vi "Auton Edit Queue.vi"(10 "Add?":bool, 11 "Delete?":bool) -> ()   [LabVIEW 2016]
uses:
  Robot Global Data.vi
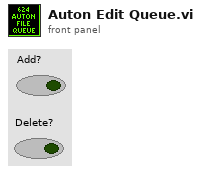
[diagram p1: front panel]
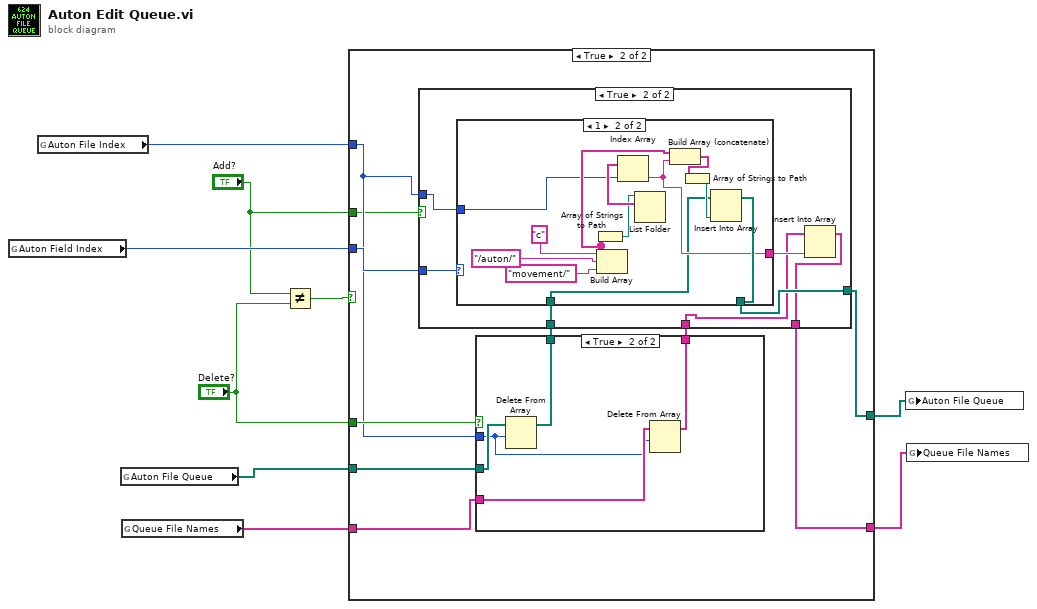
[diagram p0: block diagram]
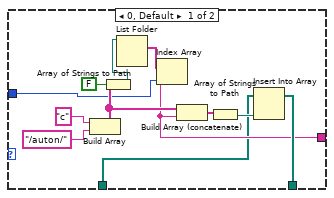
[diagram p5: hidden frame]
diagram:
  n1 = global read "Robot Global Data.vi" "Auton Field Index"() -> (w7:i32)
  n2 = global read "Robot Global Data.vi" "Auton File Index"() -> (w8:i32)
  n3 = global read "Robot Global Data.vi" "Auton File Queue"() -> (w6:path[])
  n4 = global read "Robot Global Data.vi" "Queue File Names"() -> (w5:string[])
  n5 = Not Equal?(x="Add?", y="Delete?") -> (x != y?=w9:bool)
  n6 = case shown="True" w9 {
    tunnel: w8 -> [_ w13]
    tunnel: w7 -> [_ w14]
    tunnel: [w11 w17] -> w4
    tunnel: w6 -> [w11 w21]
    tunnel: [w10 w15] -> w3
    tunnel: w5 -> [w10 w19]
    tunnel: "Delete?" -> [_ w20]
    tunnel: "Add?" -> [_ w12]
    frame False {
    }
    frame True {
      n7 = case shown="True" w20 {
        tunnel: w21 -> [w23 w28]
        tunnel: w19 -> [w22 w27]
        tunnel: [w23 w26] -> w18
        tunnel: [w22 w25] -> w16
        tunnel: w13 -> [_ w24]
        frame False {
        }
        frame True {
          n8 = Delete From Array(array=w28, length=w24) -> (array with subset deleted=w26:path[])  [unwired: 1 in, 1 out]
          n9 = Delete From Array(array=w27, length=w24) -> (array with subset deleted=w25:string[])  [unwired: 1 in, 1 out]
        }
      }
      n10 = case shown="True" w12 {
        tunnel: w18 -> [w30 w35]
        tunnel: [w30 w34] -> w17
        tunnel: w16 -> [w29 w32]
        tunnel: [w29 w31] -> w15
        tunnel: w14 -> [_ w37]
        tunnel: w13 -> [_ w36]
        frame False {
        }
        frame True {
          n11 = case shown="1" w37 {
            tunnel: [w47 w59] -> w34
            tunnel: [w40 w52] -> w33
            tunnel: w36 -> [w38 w50]
            tunnel: w35 -> [w39 w51]
            frame 0, Default {
              n12 = Build Array("c", "/auton/") -> (w42:string[])
              n13 = Array of Strings to Path(0:w42, 1:FALSE ("relative")) -> (2:w44:path)
              n14 = List Folder(path=w44) -> (filenames=w49:string[])  [unwired: 3 in, 3 out]
              n15 = Index Array(array=w49, index=w38) -> (element=w40:string)
              n16 = Build Array (concatenate)(w42, w40) -> (w41:string[])
              n17 = Array of Strings to Path(0:w41) -> (2:w48:path)  [unwired: 1 in]
              n18 = Insert Into Array(array=w39, new element=w48) -> (w47:path[])  [unwired: 1 in]
            }
            frame 1 {
              n19 = Build Array("c", "/auton/", "movement/" ("element")) -> (w54:string[])
              n20 = Array of Strings to Path(0:w54) -> (2:w55:path)  [unwired: 1 in]
              n21 = List Folder(path=w55) -> (filenames=w60:string[])  [unwired: 3 in, 3 out]
              n22 = Index Array(array=w60, index=w50) -> (element=w52:string)
              n23 = Build Array (concatenate)(w54, w52) -> (w53:string[])
              n24 = Array of Strings to Path(0:w53) -> (2:w61:path)  [unwired: 1 in]
              n25 = Insert Into Array(array=w51, new element=w61) -> (w59:path[])  [unwired: 1 in]
            }
          }
          n26 = Insert Into Array(array=w32, new element=w33) -> (w31:string[])  [unwired: 1 in]
        }
      }
    }
  }
  n27 = global write "Robot Global Data.vi" "Auton File Queue"(w4) -> ()
  n28 = global write "Robot Global Data.vi" "Queue File Names"(w3) -> ()
